vi "UI_tracking xy.vi"(7 "untracking":bool, 8 "错误输入（无错误）":errorcluster, 9 "tracking in":T4 {"centroid"."Y Centroid" format="%.2f"; "centroid"."X Centroid" format="%.2f"; "ROI Des out"."Contours"."Type" items=["No Selection", "Point", "Line", "Rectangle", "Oval", "Polygon", "Freehand Region", "Annulus", "Unused2", "Unused3", "Broken Line", "Freehand Line", "Rotated Rectangle"]}, 10 "info":T2={"data name"="", "ROI ref"=refnum, "cali ref"=refnum, "参考球？"=FALSE, "LUT"=[], "Cali array"=[], "修正次数"=2, "R_step"=0.4, "sample(quar)"=12}, 11 "image ref":T3[](array[typedef])) -> (0 "错误输出":errorcluster, 1 "xy array":cluster{"X Centroid":sgl, "Y Centroid":sgl}[](array[cluster]), 2 "tracking out":T4 {"centroid"."Y Centroid" format="%.2f"; "centroid"."X Centroid" format="%.2f"; "ROI Des out"."Contours"."Type" items=["No Selection", "Point", "Line", "Rectangle", "Oval", "Polygon", "Freehand Region", "Annulus", "Unused2", "Unused3", "Broken Line", "Freehand Line", "Rotated Rectangle"]}, 3 "radial profile array（归一化,用于LUT）":dbl[](array[numeric]), 5 "ROI Des out":T1 {"Contours"."Type" items=["No Selection", "Point", "Line", "Rectangle", "Oval", "Polygon", "Freehand Region", "Annulus", "Unused2", "Unused3", "Broken Line", "Freehand Line", "Rotated Rectangle"]})   [LabVIEW 2017]
doc: "本VI 利用QI算法计算XY的实时位置并进行ROI追踪，其中布尔输入tracking 为否时，ROI不进行追踪，此时可以手动移动ROI，tracking 布尔按钮与暂停测量联动，即不追踪时也不记录数据。"
uses:
  <vilib>/vision/Image Controls.llb/IMAQ Image.ctl
  control/Bead track.ctl
  control/bead info.ctl
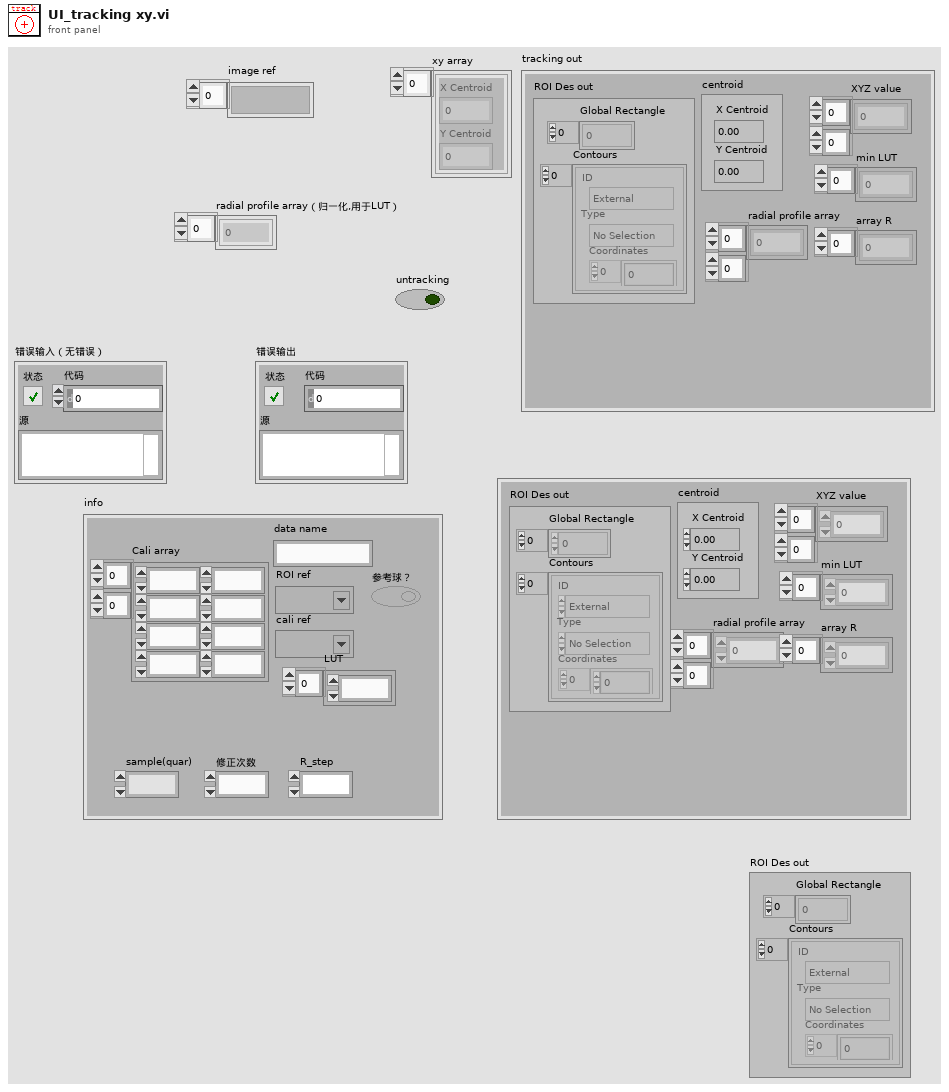
[diagram p1: front panel]
types:
  T1 = typedef "ROI Descriptor" = cluster{"Global Rectangle":i32[], "Contours":cluster{"ID":enum32{"External", "Internal"}, "Type":u32, "Coordinates":i32[]}[]}
  T2 = typedef "bead info.ctl" = cluster{"data name":string, "ROI ref":T3, "cali ref":T3, "参考球？":bool, "LUT":dbl[], "Cali array":dbl[][], "修正次数":i32, "R_step":dbl, "sample(quar)":i32}
  T3 = typedef "IMAQ Image.ctl" = refnum<image>
  T4 = typedef "Bead track.ctl" = cluster{"XYZ value":dbl[][], "radial profile array":dbl[][], "min LUT":dbl[], "ROI Des out":T1, "array R":dbl[], "centroid":cluster{"X Centroid":sgl, "Y Centroid":sgl}}
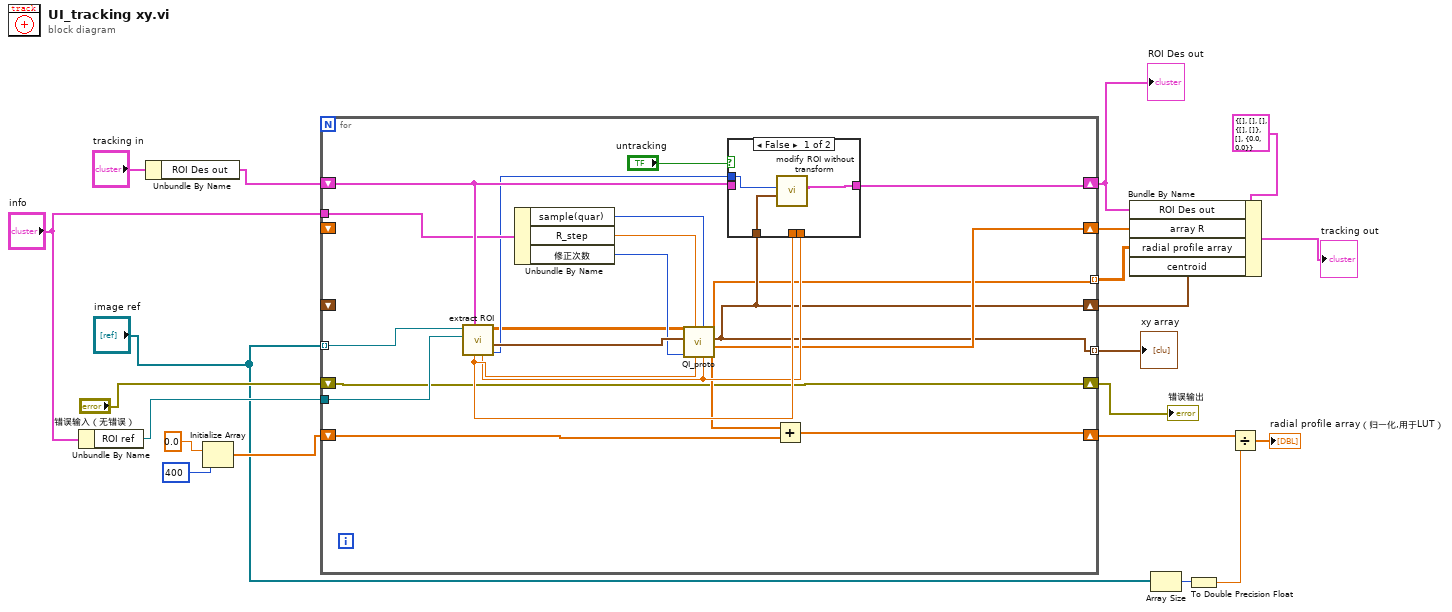
[diagram p0: block diagram]
diagram:
  n1 = Unbundle By Name("info") -> ("ROI ref"=w10:T3)
  n2 = Unbundle By Name("tracking in") -> ("ROI Des out"=w15:T1)
  n3 = Initialize Array(0.0 ("元素"), 400 ("维数大小")) -> (w17:dbl[])
  n4 = for "For循环" {
    shift-right: [w38] -> w7
    shift-left: w17 -> [w26]
    shift-right: [w36] -> w4
    shift-left: w15 -> [w37]
    shift-right: [w24] -> w1
    shift-left: "错误输入（无错误）" -> [w24]
    tunnel: w10 -> [w35]
    tunnel: "info" -> [w34]
    tunnel: "image ref" -> [w30] mode=indexing
    tunnel: [w27] -> w9 mode=indexing
    tunnel: [w28] -> w8 mode=indexing
    shift-right: [w29] -> w3
    shift-left: _ -> [_]
    shift-right: [w28] -> w2
    shift-left: _ -> [_]
    n5 = call "extract ROI.vi"("ROI Descriptor"=w37, "ROI ref in"=w35, "CCD image ref"=w30) -> ("ROI SIZE"=w23:i32, "Centroid XY"=w39:cluster{"X Centroid":sgl, "Y Centroid":sgl}, "img_out"=w22:dbl[][], "Y_base"=w40:sgl, "X_base"=w41:sgl)  [unwired: 4 in]
    n6 = Unbundle By Name(w34) -> ("sample(quar)"=w31:i32, "R_step"=w32:dbl, "修正次数"=w33:i32)
    n7 = call "QI_proto.vi"("Y_base"=w40, "sample(quar)"=w31, "X_base"=w41, "R_step"=w32, "修正次数"=w33, "Centroid"=w39, "ROI array"=w22) -> ("array R"=w29:dbl[], "xc and yc"=w28:cluster{"X Centroid":sgl, "Y Centroid":sgl}, "radial profile array"=w27:dbl[])  [unwired: 2 in]
    n8 = case shown="False" "untracking" {
      tunnel: w41 -> [_ _]
      tunnel: w40 -> [_ _]
      tunnel: w37 -> [_ w45]
      tunnel: [w43 w45] -> w36
      tunnel: w28 -> [w44 _]
      tunnel: w23 -> [w42 _]
      frame False {
        n9 = call "modify ROI without transform.vi"("new x y"=w44, "ROI size"=w42) -> ("ROI Descriptor out"=w43:T1)  [unwired: 8 in, 1 out]
      }
      frame True {
      }
    }
    n10 = Add(x=w27, y=w26) -> (x+y=w38:dbl[])
  }
  "错误输出" <- w1
  "xy array" <- w8
  "ROI Des out" <- w4
  n11 = Bundle By Name(cluster=T4 {"XYZ value"=[], "radial profile array"=[], "min LUT"=[], "ROI Des out"={"Global Rectangle"=[], "Contours"=[]}, "array R"=[], "centroid"={"X Centroid"=0.0, "Y Centroid"=0.0}} ("tracking"), "ROI Des out"=w4, "array R"=w3, "radial profile array"=w9, "centroid"=w2) -> (→"tracking out":T4)
  n12 = Array Size(array="image ref") -> (size(s)=w20:i32)
  n13 = To Double Precision Float(number=w20) -> (double precision float=w19:dbl)
  n14 = Divide(x=w7, y=w19) -> (x/y=→"radial profile array（归一化,用于LUT）":dbl[])
